vi "SingleShot_Label Localization.vi"() -> (2 "localized control labels":string[](array[string]), 3 "DNL_unlocalized control labels":string[](array[string]), 4 "DNL_unlocalized string constant labels":string[](array[string]), 6 "localized string constant values":string[](array[string]))   [LabVIEW 2022 SP3]
panel:
  in  "static localized string constant values":string[](array[string])=["Signal Statistics:\\n Mean: %0.3f", "Time", "Amplitude", "Text File", "LabVIEW TDMS File", "Data acquired.", "Data not acquired.", "Data loaded.", "Data not loaded.", "Data saved.", "Data not saved.", "Data exported.", "Data not exported.", "Stopped."]
  in  "static localized control labels":string[](array[string])
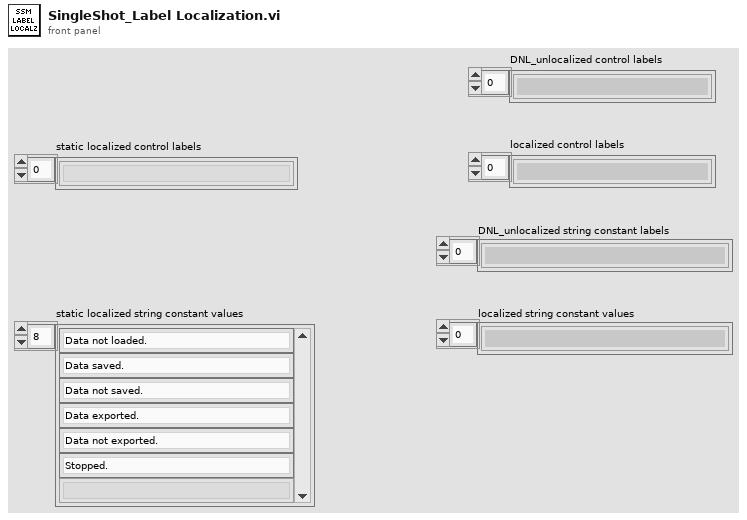
[diagram p1: front panel]
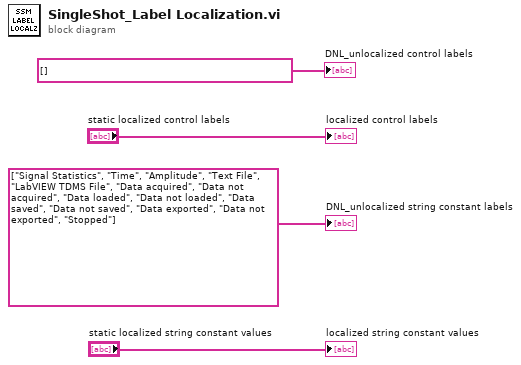
[diagram p0: block diagram]
diagram:
  "DNL_unlocalized control labels" <- string[] [] ("DNL_unlocalized control labels")
  "localized control labels" <- "static localized control labels"
  "localized string constant values" <- "static localized string constant values"
  "DNL_unlocalized string constant labels" <- string[] ["Signal Statistics", "Time", "Amplitude", "Text File", "LabVIEW TDMS File", "Data acquired", "Data not acquired", "Data loaded", "Data not loaded", "Data saved", "Data not saved", "Data exported", "Data not exported", "Stopped"] ("DNL_unlocalized control labels")
